vi "RT_Velocity mode_Oct 25_R4.vi"() -> ()   [LabVIEW 2018]
uses:
  Type Defs/BL Measurement States.ctl
  <vilib>/Platform/TimedLoop/XDataNode/timing_clust.ctl
  <vilib>/Platform/TimedLoop/XDataNode/nitl_modes.ctl
  <vilib>/Platform/TimedLoop/XDataNode/wakeup.ctl
  <vilib>/FPGAPlugInAG/myRIO-1900/niLvFpga_Open_myRIO-1900.vi
  <vilib>/rvi/interface/common/dynamic/niFpgaDynamicAddResources.vi
  <vilib>/Utility/error.llb/Error Cluster From Error Code.vi
  <vilib>/rvi/errors/niLvFpgaAdjustHostInterfaceError.vi
  <vilib>/FPGAPlugInAG/Dynamic/niLvFpga_Close_Dynamic.vi
  <vilib>/Platform/TimedLoop/XDataNode/XDataNode.xnode
  <vilib>/rvi/interface/nirviOpenFPGA/nirviOpenFPGA.xnode
  UNCC Watt balance Oct19/FPGA Bitfiles/UNCCWattbalanceO_FPGATarget_fpganestedFORW&R_aHmrZ4eE-L4.lvbitx
  FPGA files/fpga_nestedFOR_W&R_ADC_W_2DACs_Write_then_CLK.vi
  <vilib>/rvi/interface/nirviReadWriteControl/nirviReadWriteControl.xnode
  <vilib>/rvi/interface/nirviCloseFPGA/nirviCloseFPGA.xnode
  <vilib>/Platform/TimedLoop/XDataNode/XDNodeRunTimeDep.lvlib
  NiFpgaLv.dll
  <vilib>/rvi/interface/Simulation/niFpgaSimulationCallBeginRW.vi
panel:
  in  "threshold valleys":dbl=0.5
  in  "threshold peaks":dbl=-0.5
  in  "offset (V)":dbl
  in  "loop period (us)":i64=200
  in  "frequ (Hz)":dbl=30.0
  in  "amplitude (V)":dbl format="%.1f"
  out "N":i32=1
  out "avg BL (V/m/s)":dbl=14.560128714838308 format="%.2g"
  out "raw BL (V/m/s)":dbl=14.560128714838308 format="%.2f"
  in  "BL meas type":bool=TRUE
  in  "Reset BL":bool
  in  "Measure BL":bool
  in  "Stop Button":bool
  in  "no. data points":u16=500
  out "?":cluster{dbl, dbl}(graph)={-2.3587286570944648, 2.2359199005204733}
  out "Lissajou":cluster{dbl[], dbl[]}(graph) caption="XY Graph - dark"
  out "Queue On":bool
  out "Late":bool
  # "COIL CONTROL"
  # "MEASURED BL VALUES"
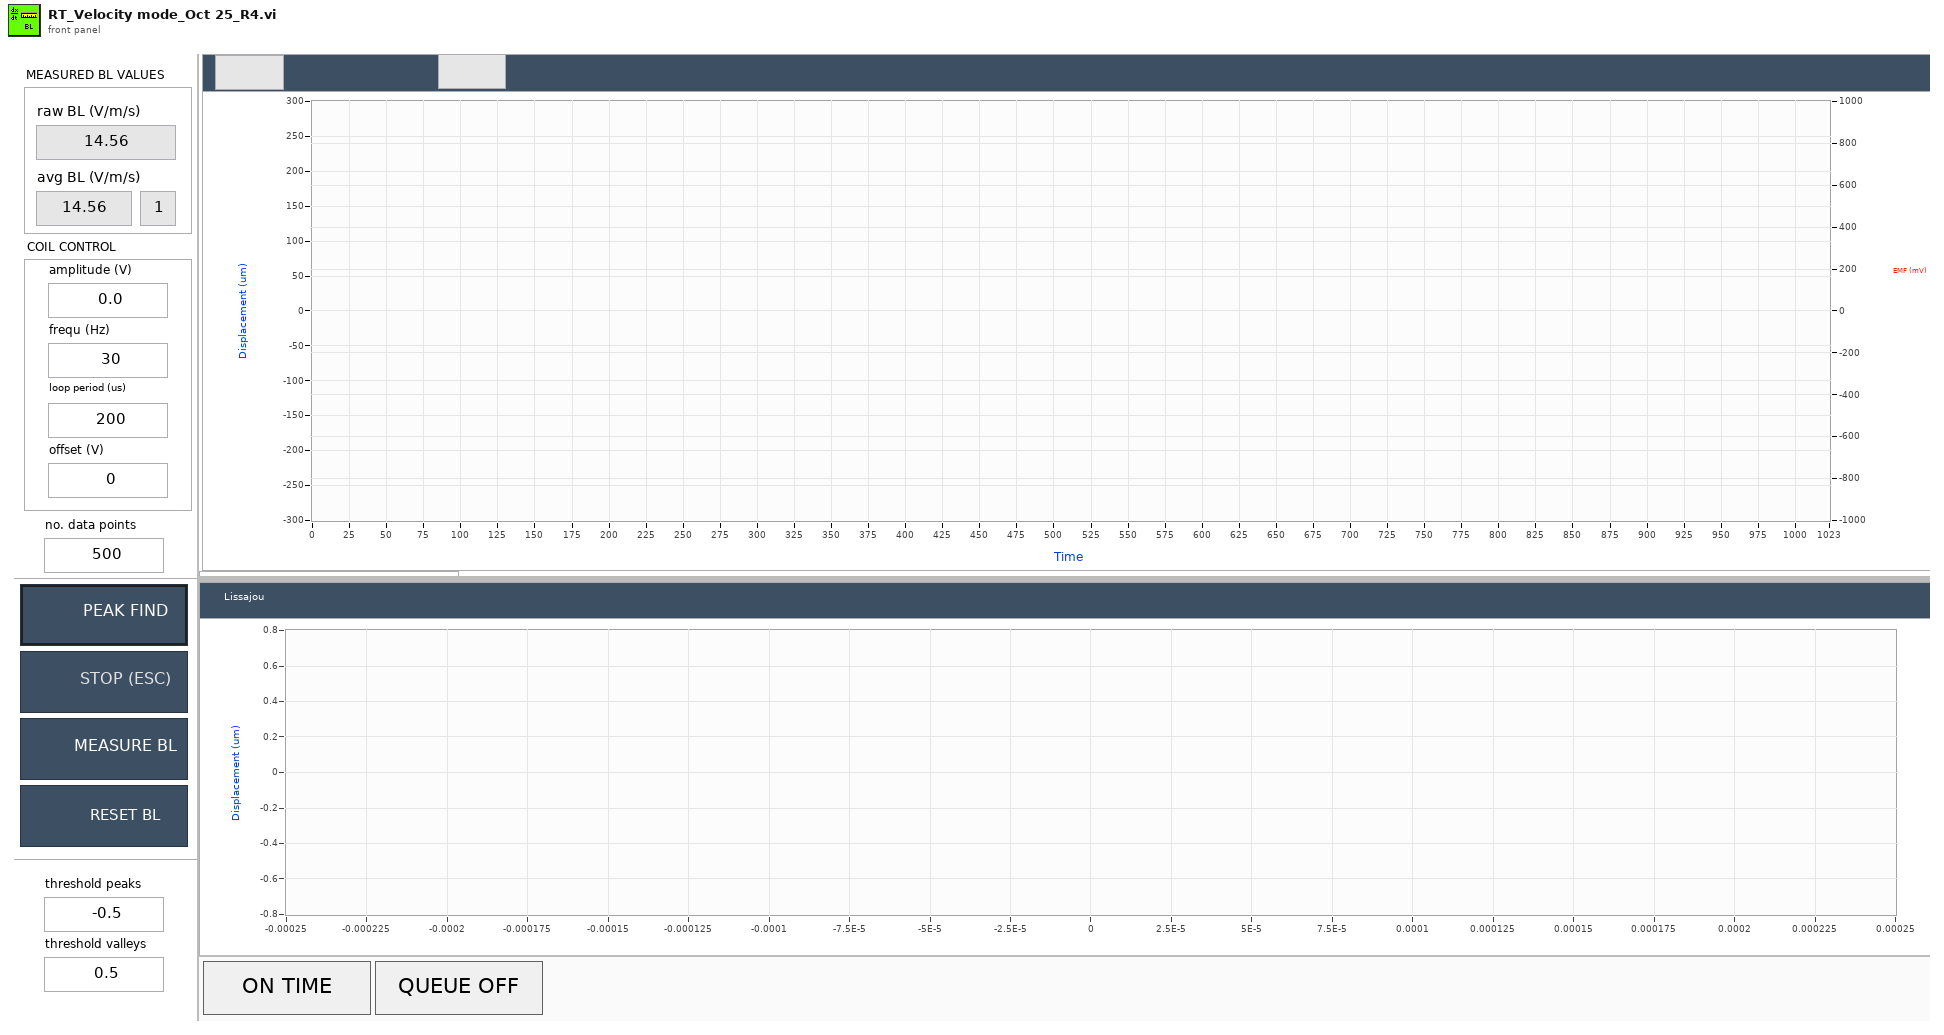
[diagram p1: front panel]
types:
  T1 = typedef "BL Measurement States.ctl" = enum16{"reset BL avg", "idle", "initialize", "collect data", "prepare data", "fit sine", "exit meas"}
  T2 = typedef "XDNodeRunTimeDep.lvlib/timing_clust.ctl" = cluster{"Expected End [f-1]":u64, "Actual End [f-1]":u64, "Finished Late? [f-1]":bool, "Expected End [i-1]":u64, "Actual End [i-1]":u64, "Finished Late? [i-1]":bool, "Expected Start [i]":u64, "Actual Start [i]":u64, "Expected Start [f]":u64, "Actual Start [f]":u64, "Source Name":string, "Structure Name":string, "Period":i64, "Deadline":i64, "Offset":i64, "Start":i64, "Priority":i32, "Timeout":i32, "Mode":T3, "Wakeup Reason":T4, "Error":errorcluster, "Source Type":string, "Secondary Source Type":string, "Global End Time":u64, "Global Start Time":u64, "Frame Duration":u64, "Iteration Duration":u64, "Assigned CPU":i32, "I/O Scan Engine Mode":u32}
  T3 = typedef "XDNodeRunTimeDep.lvlib/nitl_modes.ctl" = enum32{"No Change", "Process missed periods, maintain original phase", "Discard missed periods, maintain original phase", "Process missed periods, ignore original phase", "Discard missed periods, ignore original phase"}
  T4 = typedef "XDNodeRunTimeDep.lvlib/wakeup.ctl" = enum32{"Normal", "Aborted", "Asynchronous wakeup", "Timing source error", "Timed loop error", "Timeout"}
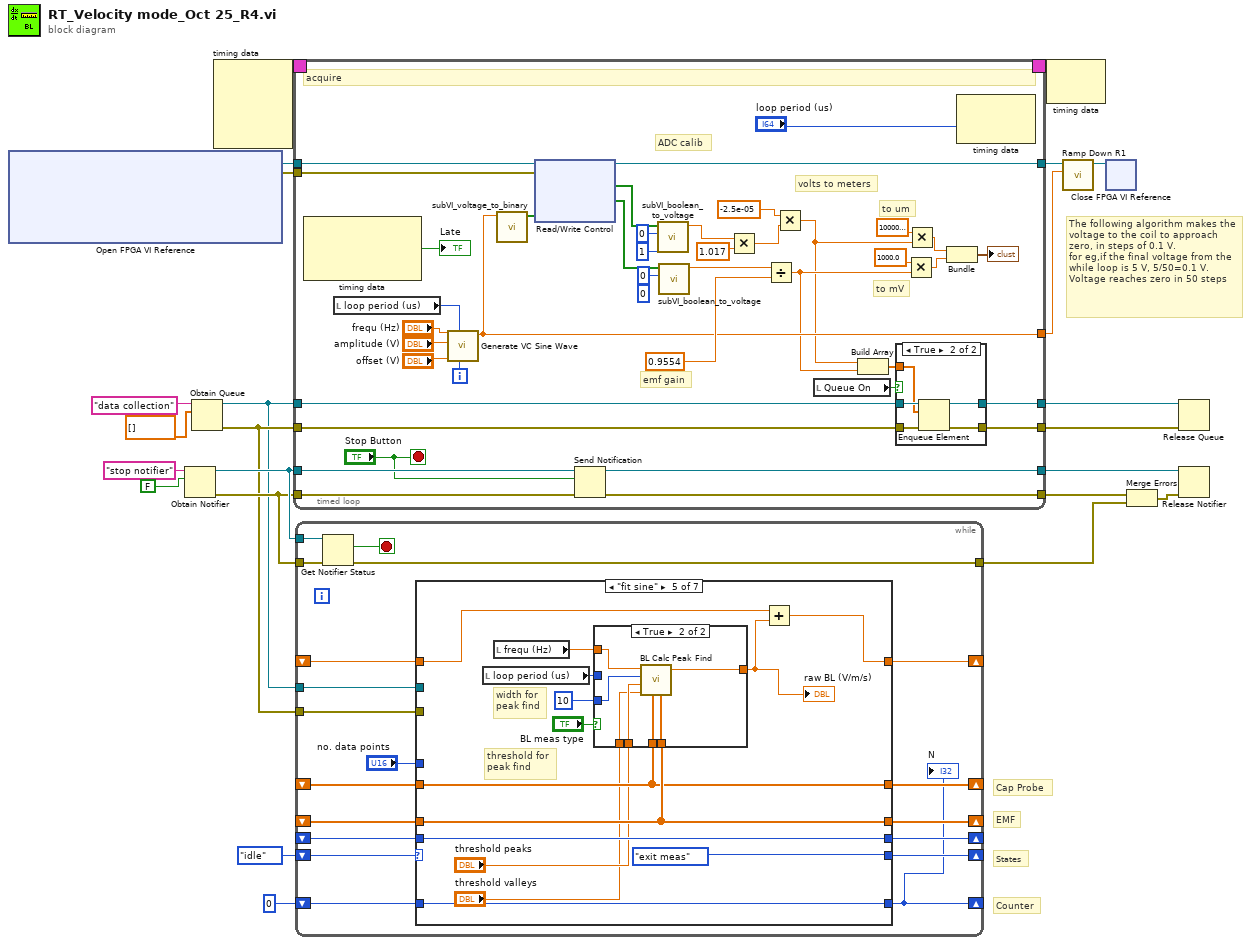
[diagram p0: block diagram]
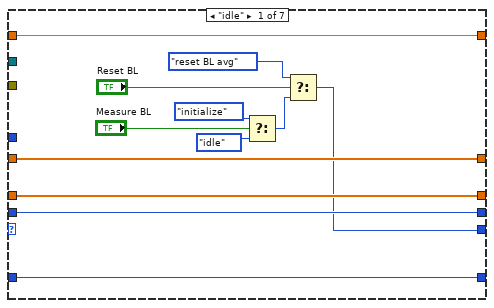
[diagram p2: hidden frame]
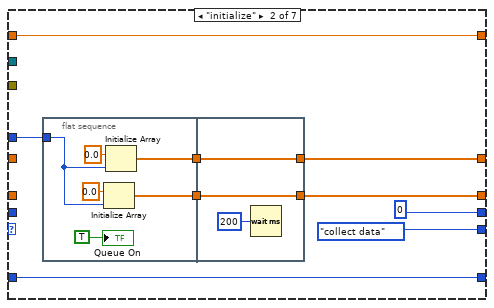
[diagram p3: hidden frame]
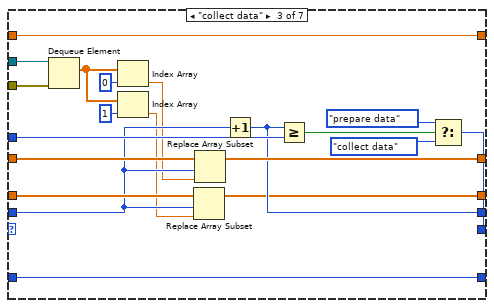
[diagram p4: hidden frame]
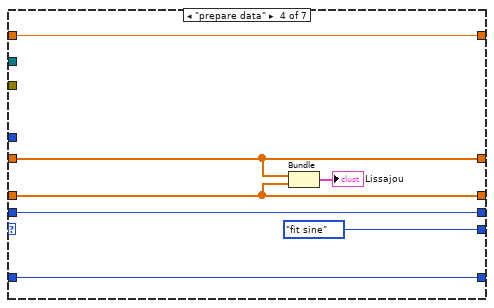
[diagram p5: hidden frame]
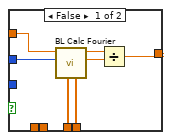
[diagram p6: hidden frame]
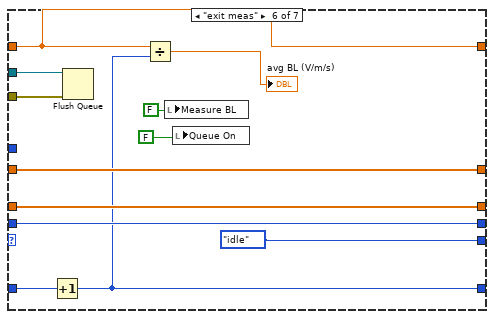
[diagram p7: hidden frame]
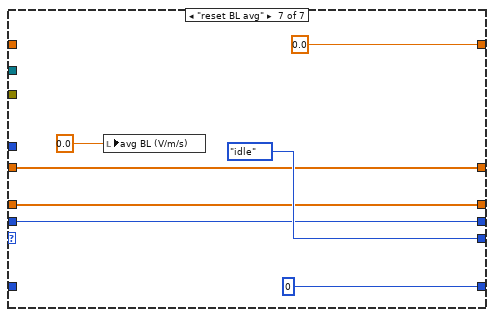
[diagram p8: hidden frame]
diagram:
  # "The following algorithm makes the voltage to the coil to approach zero, in steps of 0.1 V.\nfor eg,if the final voltage from the while loop is 5 V, 5/50=0.1 V. Voltage reaches zero in 50 steps"
  # "States"
  # "Counter"
  # "EMF"
  # "Cap Probe"
  n1 = xnode "Open FPGA VI Reference"() -> ("FPGA VI Reference Out"=w21:refnum<k20>, "error out"=w20:errorcluster)  [unwired: 2 in]
  n2 = Obtain Notifier(name (unnamed)="stop notifier", notification data type=FALSE) -> (notifier out=w12:refnum<notifier>, error out=w11:errorcluster)  [unwired: 2 in, 1 out]
  n3 = Obtain Queue(name (unnamed)="data collection", element data type=dbl[] [] ("appended array")) -> (queue out=w1:refnum<queue>, error out=w2:errorcluster)  [unwired: 3 in, 1 out]
  n4 = node-c288() -> (w23:T2)  [unwired: 4 in]
  n5 = timed-loop {
    timing: w23 -> [_]
    timing-out: [_] -> w22
    tunnel: w21 -> [w49]
    tunnel: w20 -> [w58]
    tunnel: [w50] -> w17
    tunnel: [w36] -> w18
    tunnel: w12 -> [w48]
    tunnel: w11 -> [w46]
    tunnel: [w45] -> w7
    tunnel: [w44] -> w10
    tunnel: w1 -> [w42]
    tunnel: w2 -> [w41]
    tunnel: [w39] -> w4
    tunnel: [w38] -> w3
    i -> [w64]
    stop <- "Stop Button" stop-if-true
    (unwired) i16 0 ("Gain")
    # "emf gain"
    # "ADC calib"
    # "to mV"
    # "to um"
    # "volts to meters"
    # "acquire"
    n6 = node-c288() -> (→"Late":bool)  [unwired: 1 in, 2 out]
    n7 = local read "loop period (us)"() -> (w62:i64)
    n8 = call "Generate VC Sine Wave.vi"("Counter"=w64, "Period (us)"=w62, "offset (V)"="offset (V)", "amplitude (V)"="amplitude (V)", "frequency (kHz)"="frequ (Hz)") -> ("V"=w50:dbl)  [unwired: 6 in]
    n9 = call "subVI_voltage_to_binary.vi"("voltage"=w50) -> ("binary"=w59:bool[])  [unwired: 10 in]
    n10 = xnode "Read/Write Control"("FPGA VI Reference In"=w49, "error in"=w58, "DAC 1 write"=w59) -> ("FPGA VI Reference Out"=w36:refnum<k20>, "ADC  1 R"=w54:bool[], "ADC 2 R"=w53:bool[])  [unwired: 1 out]
    n11 = Send Notification(notification="Stop Button", notifier=w48, error in (no error)=w46) -> (notifier out=w45:refnum<notifier>, error out=w44:errorcluster)
    n12 = call "subVI_boolean_to_voltage.vi"("Gain"=i16 1, "UNI"=i16 0, "ADC read"=w54) -> ("V"=w34:dbl)  [unwired: 8 in]
    n13 = call "subVI_boolean_to_voltage.vi"("UNI"=i16 0, "ADC read"=w53) -> ("V"=w52:dbl)  [unwired: 9 in]
    n14 = Multiply(x=w34, y=1.017) -> (x*y=w32:dbl)
    n15 = Divide(x=w52, y=0.9554 ("EMF Gain")) -> (x/y=w43:dbl)
    n16 = Multiply(x=-2.5e-05, y=w32) -> (x*y=w30:dbl)
    n17 = local read "Queue On"() -> (w37:bool)
    n18 = Build Array(w30, w43) -> (w40:dbl[])
    n19 = case shown="True" w37 {
      tunnel: w42 -> [w66 w71]
      tunnel: w41 -> [w65 w70]
      tunnel: w40 -> [_ w69]
      tunnel: [w66 w68] -> w39
      tunnel: [w65 w67] -> w38
      frame False {
      }
      frame True {
        n20 = Enqueue Element(queue=w71, element=w69, error in (no error)=w70) -> (queue out=w68:refnum<queue>, error out=w67:errorcluster)  [unwired: 1 in, 1 out]
      }
    }
    n21 = Multiply(x=1000.0, y=w43) -> (x*y=w51:dbl)
    n22 = Multiply(x=1000000.0, y=w30) -> (x*y=w31:dbl)
    n23 = Bundle(w31, w51) -> (→"?":cluster{dbl, dbl})  [unwired: 1 in]
    n24 = node-c288("loop period (us)") -> ()  [unwired: 1 in, 1 out]
  }
  n25 = while {
    shift-right: [w77] -> _
    shift-left: 0 -> [w86]
    shift-right: [w90] -> _
    shift-left: _ -> [w87]
    shift-right: [w91] -> _
    shift-left: _ -> [w88]
    shift-right: [w92] -> _
    shift-left: _ -> [w89]
    shift-right: [w94] -> _
    shift-left: _ -> [w95]
    shift-right: [w93] -> _
    shift-left: BL_Measurement_States."idle" ("BL meas states") -> [w80]
    tunnel: w12 -> [w84]
    tunnel: w11 -> [w83]
    tunnel: [w81] -> w9
    tunnel: w2 -> [w78]
    tunnel: w1 -> [w79]
    stop <- w82 stop-if-true
    n26 = Get Notifier Status(notifier=w84, error in (no error)=w83) -> (current notification=w82:bool, error out=w81:errorcluster)  [unwired: 3 out]
    n27 = case shown="\"fit sine\"" w80 {
      tunnel: [w100 BL_Measurement_States."collect data" ("BL meas states") w139 BL_Measurement_States."fit sine" ("BL meas states") BL_Measurement_States."exit meas" ("BL meas states") BL_Measurement_States."idle" ("BL meas states") BL_Measurement_States."idle" ("BL meas states")] -> w93
      tunnel: [w104 w114 w140 w148 w160 w191 w198] -> w92
      tunnel: [w103 w113 w136 w146 w164 w188 w197] -> w91
      tunnel: w89 -> [w104 _ w142 w148 w160 w191 w198]
      tunnel: w87 -> [w105 _ w135 w152 w166 w190 w196]
      tunnel: [w105 0 w138 w152 w166 w190 w196] -> w90
      tunnel: "no. data points" -> [_ w112 w141 _ _ _ _]
      tunnel: w88 -> [w103 _ w137 w146 w164 w188 w197]
      tunnel: [w98 w111 w134 w150 w157 w187 0.0] -> w94
      tunnel: w95 -> [w98 w111 w134 w150 w163 w187 _]
      tunnel: w86 -> [w99 w110 w133 w149 w162 w182 _]
      tunnel: [w99 w110 w133 w149 w162 w181 0] -> w77
      tunnel: w79 -> [_ _ w132 _ _ w186 _]
      tunnel: w78 -> [_ _ w131 _ _ w185 _]
      frame "idle" {
        n28 = Select(t=BL_Measurement_States."initialize" ("BL meas states"), s="Measure BL", f=BL_Measurement_States."idle" ("BL meas states 2")) -> (s? t:f=w101:T1)
        n29 = Select(t=BL_Measurement_States."reset BL avg" ("BL meas states"), s="Reset BL", f=w101) -> (s? t:f=w100:T1)
      }
      frame "initialize" {
        n30 = flat-sequence {
          tunnel: w112 -> [w120]
          tunnel: [w122] -> w109
          tunnel: [w121] -> w108
          tunnel: [w124] -> w113
          tunnel: [w125] -> w114
          tunnel: w109 -> [w125]
          tunnel: w108 -> [w124]
          frame #0 {
            n31 = Initialize Array(0.0 ("element"), w120) -> (w121:dbl[])
            n32 = Initialize Array(0.0 ("element"), w120) -> (w122:dbl[])
            "Queue On" <- TRUE
          }
          frame #1 {
            n33 = Wait (ms)(milliseconds to wait=u32 200) -> ()  [unwired: 1 out]
          }
        }
      }
      frame "collect data" {
        n34 = Dequeue Element(queue=w132, error in (no error)=w131) -> (element=w130:dbl[])  [unwired: 1 in, 3 out]
        n35 = Index Array(array=w130, index=0) -> (element=w127:dbl)
        n36 = Index Array(array=w130, index=1) -> (element=w126:dbl)
        n37 = Replace Array Subset(array=w137, new element=w126, index=w135) -> (w136:dbl[])
        n38 = Replace Array Subset(array=w142, new element=w127, index=w135) -> (w140:dbl[])
        n39 = Increment(x=w135) -> (x+1=w138:i32)
        n40 = Greater Or Equal?(x=w138, y=w141) -> (x >= y?=w143:bool)
        n41 = Select(t=BL_Measurement_States."prepare data" ("BL meas states"), s=w143, f=BL_Measurement_States."collect data" ("BL meas states 2")) -> (s? t:f=w139:T1)
      }
      frame "prepare data" {
        n42 = Bundle(w148, w146) -> (→"Lissajou":cluster{dbl[], dbl[]})  [unwired: 1 in]
      }
      frame "fit sine" {
        # "threshold for\npeak find"
        # "width for\npeak find"
        n43 = local read "loop period (us)"() -> (w161:i64)
        n44 = local read "frequ (Hz)"() -> (w159:dbl)
        n45 = case shown="True" "BL meas type" {
          tunnel: w164 -> [w168 w176]
          tunnel: w161 -> [w173 _]
          tunnel: w160 -> [w167 w180]
          tunnel: w159 -> [w172 w179]
          tunnel: 10 ("width") -> [_ w178]
          tunnel: [w171 w177] -> w155
          tunnel: "threshold peaks" -> [_ w175]
          tunnel: "threshold valleys" -> [_ w174]
          frame False {
            n46 = call "BL Calc Fourier.vi"("EMF"=w168, "cap probe"=w167, "Period (us)"=w173, "FREQU"=w172) -> ("velocity"=w169:dbl, "EMF"=w170:dbl)  [unwired: 6 in]
            n47 = Divide(x=w170, y=w169) -> (x/y=w171:dbl)
          }
          frame True {
            n48 = call "BL Calc Peak Find.vi"("back emf"=w176, "cap probe"=w180, "threshold valleys"=w174, "threshold peaks"=w175, "width"=w178, "frequency (Hz)"=w179) -> ("Numeric"=w177:dbl)  [unwired: 5 in]
          }
        }
        "raw BL (V/m/s)" <- w155
        n49 = Add(x=w163, y=w155) -> (x+y=w157:dbl)
      }
      frame "exit meas" {
        n50 = Increment(x=w182) -> (x+1=w181:i32)
        n51 = Flush Queue(queue=w186, error in (no error)=w185) -> ()  [unwired: 3 out]
        n52 = Divide(x=w187, y=w181) -> (x/y=→"avg BL (V/m/s)":dbl)
        n53 = local write "Measure BL"(FALSE) -> ()
        n54 = local write "Queue On"(FALSE) -> ()
      }
      frame "reset BL avg" {
        n55 = local write "avg BL (V/m/s)"(0.0 ("BL")) -> ()
      }
    }
    "N" <- w77
  }
  n56 = node-c288(w22) -> ()  [unwired: 1 out]
  n57 = call "Ramp Down R1.vi"("V"=w17, "Refnum in"=w18) -> ("Refnum out"=w19:refnum<k20>)  [unwired: 9 in]
  n58 = xnode "Close FPGA VI Reference"("FPGA VI Reference In"=w19) -> ()  [unwired: 1 in, 1 out]
  n59 = Merge Errors(w10, w9) -> (w8:errorcluster)
  n60 = Release Queue(queue=w4, error in (no error)=w3) -> ()  [unwired: 1 in, 3 out]
  n61 = Release Notifier(notifier=w7, error in (no error)=w8) -> ()  [unwired: 1 in, 3 out]
